vi "Get Channel Name Core.vi"(8 "error in (no error)":errorcluster, 10 "Channel Index (1)":i32=1, 11 "IVI_Scope in":refnum<class "IVI_Scope.lvclass">) -> (0 "error out":errorcluster, 2 "Channel Name":string, 3 "IVI_Scope out":refnum<class "IVI_Scope.lvclass">)   [LabVIEW 2015, in "IVI_Scope.lvlib" / "IVI_Scope.lvclass"]
doc: "This VI returns the highest-level channel name that corresponds to the specific driver channel string that is in the channel table at an index you specify."
uses:
  IVI_Scope.lvclass
  IVI_Scope.lvclass/IVI_Scope.ctl
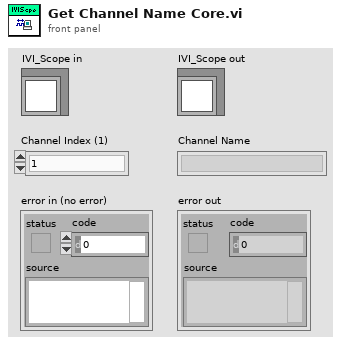
[diagram p1: front panel]
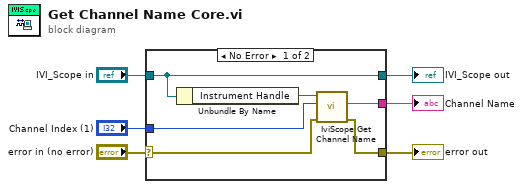
[diagram p0: block diagram]
diagram:
  n1 = case shown="No Error" "error in (no error)" {
    selector: "error in (no error)" -> [w10 w14]
    tunnel: [w9 w14] -> w5
    tunnel: [w12 w13] -> w3
    tunnel: "IVI_Scope in" -> [w12 w13]
    tunnel: "Channel Index (1)" -> [w8 _]
    tunnel: [w7 _] -> w1
    frame No Error {
      n2 = Unbundle By Name(w12) -> ("Instrument Handle"=w11:refnum<k15>)
      n3 = call <vilib>:"IviScope Get Channel Name.vi"("error in (no error)"=w10, "Channel Index (1)"=w8, "instrument handle"=w11) -> ("error out"=w9:errorcluster, "Channel Name"=w7:string)  [unwired: 6 in, 1 out]
    }
    frame Error {
    }
  }
  "error out" <- w5
  "IVI_Scope out" <- w3
  "Channel Name" <- w1
